vi "Read Asynchronous_.vi"(8 "error in":errorcluster, 11 "Module Editor Node in":refnum<class "module editor node.lvclass">) -> (0 "error out":errorcluster, 2 "Asynchronous?":bool, 3 "Module Editor Node out":refnum<class "module editor node.lvclass">)   [LabVIEW 2013, in "PL Framework Configuration Tool.lvlib" / "module editor node.lvclass"]
uses:
  module editor node.lvclass
  module editor node.lvclass/module editor node.ctl
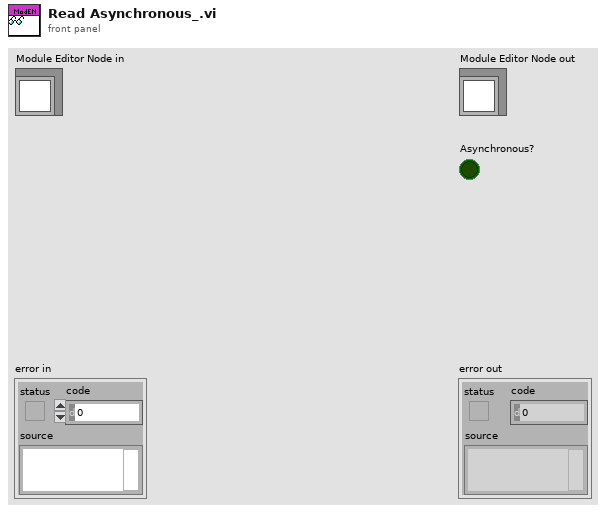
[diagram p1: front panel]
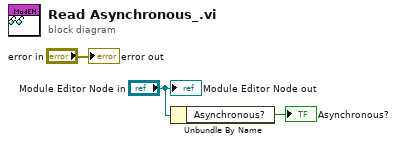
[diagram p0: block diagram]
diagram:
  n1 = Unbundle By Name("Module Editor Node in") -> ("Asynchronous?"=→"Asynchronous?":bool)
  "error out" <- "error in"
  "Module Editor Node out" <- "Module Editor Node in"
